vi "Graph vindu settinger.vi"(1 "Action(GET)":enum16{"GET", "SET"}(ring), 7 "Settigner fra MAin in":T1 {"Plot  L1"."Line Width" items=["0", "1", "2", "3", "4", "5"]; "Plot  L1"."Var Tag" items=["", "Wire Length", "Wire Tension", "Wire Speed", "Topside Voltage", "Tool Head Voltage", "Current", "Resistance"]; "Plot  L2"."Line Width" items=["0", "1", "2", "3", "4", "5"]; "Plot  L2"."Var Tag" items=["", "Wire Length", "Wire Tension", "Wire Speed", "Topside Voltage", "Tool Head Voltage", "Current", "Resistance"]; "Plot  R1"."Line Width" items=["0", "1", "2", "3", "4", "5"]; "Plot  R1"."Var Tag" items=["", "Wire Length", "Wire Tension", "Wire Speed", "Topside Voltage", "Tool Head Voltage", "Current", "Resistance"]; "Plot  R2"."Line Width" items=["0", "1", "2", "3", "4", "5"]; "Plot  R2"."Var Tag" items=["", "Wire Length", "Wire Tension", "Wire Speed", "Topside Voltage", "Tool Head Voltage", "Current", "Resistance"]}, 11 "error in (no error)":errorcluster) -> (8 "Settigner fra MAin out":T1 {"Plot  L1"."Line Width" items=["0", "1", "2", "3", "4", "5"]; "Plot  L1"."Var Tag" items=["", "Wire Length", "Wire Tension", "Wire Speed", "Topside Voltage", "Tool Head Voltage", "Current", "Resistance"]; "Plot  L2"."Line Width" items=["0", "1", "2", "3", "4", "5"]; "Plot  L2"."Var Tag" items=["", "Wire Length", "Wire Tension", "Wire Speed", "Topside Voltage", "Tool Head Voltage", "Current", "Resistance"]; "Plot  R1"."Line Width" items=["0", "1", "2", "3", "4", "5"]; "Plot  R1"."Var Tag" items=["", "Wire Length", "Wire Tension", "Wire Speed", "Topside Voltage", "Tool Head Voltage", "Current", "Resistance"]; "Plot  R2"."Line Width" items=["0", "1", "2", "3", "4", "5"]; "Plot  R2"."Var Tag" items=["", "Wire Length", "Wire Tension", "Wire Speed", "Topside Voltage", "Tool Head Voltage", "Current", "Resistance"]}, 15 "error out":errorcluster)   [LabVIEW 2011]
uses:
  Settigner fra Main.ctl
  Graph/Plot selector.ctl
  Graph/Y scale cluster.ctl
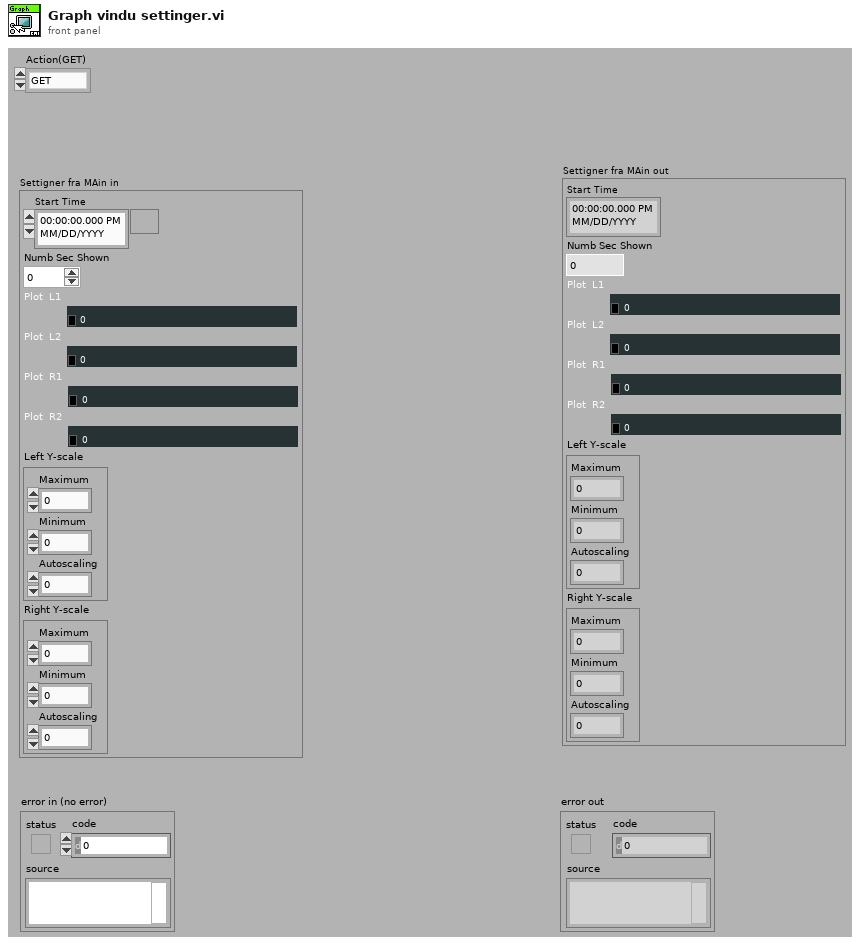
[diagram p1: front panel]
types:
  T1 = typedef "Settigner fra Main.ctl" = cluster{"Start Time":timestamp, "Numb Sec Shown":i32, "Plot  L1":T2, "Plot  L2":T2, "Plot  R1":T2, "Plot  R2":T2, "Left Y-scale":T3, "Right Y-scale":T3}
  T2 = typedef "Plot selector.ctl" = cluster{"Var Tag":u16, "Color":u32, "Line Width":u16}
  T3 = typedef "Y scale cluster.ctl" = cluster{"Maximum":dbl, "Minimum":dbl, "Autoscaling":i32}
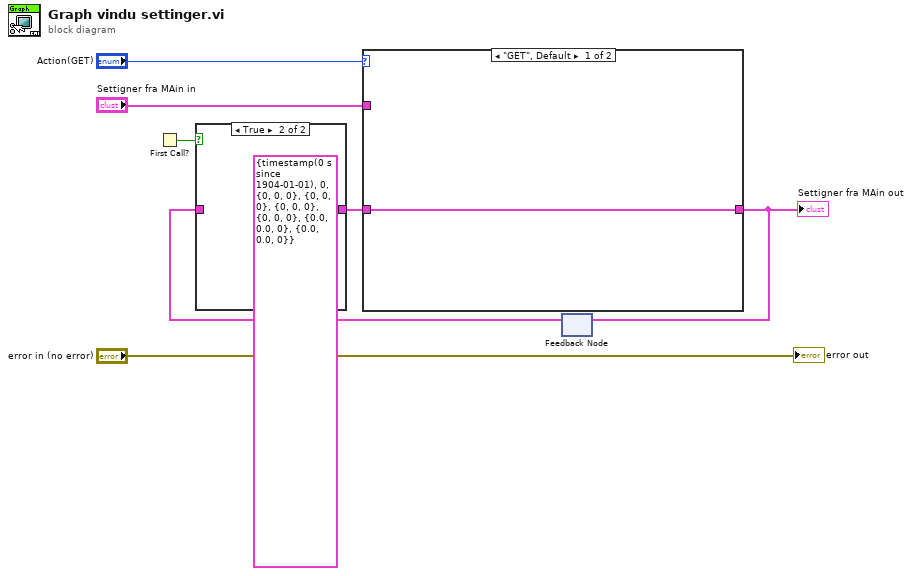
[diagram p0: block diagram]
diagram:
  n1 = First Call?() -> (First Call?: T/F=w4:bool)
  n2 = feedback #1() -> (w5:T1)  [unwired: 1 in]
  n3 = case shown="True" w4 {
    tunnel: w5 -> [w8 _]
    tunnel: [w8 T1 {"Start Time"=timestamp(0 s since 1904-01-01), "Numb Sec Shown"=0, "Plot  L1"={"Var Tag"=0, "Color"=0, "Line Width"=0}, "Plot  L2"={"Var Tag"=0, "Color"=0, "Line Width"=0}, "Plot  R1"={"Var Tag"=0, "Color"=0, "Line Width"=0}, "Plot  R2"={"Var Tag"=0, "Color"=0, "Line Width"=0}, "Left Y-scale"={"Maximum"=0.0, "Minimum"=0.0, "Autoscaling"=0}, "Right Y-scale"={"Maximum"=0.0, "Minimum"=0.0, "Autoscaling"=0}} ("Settigner fra MAin")] -> w2
    frame False {
    }
    frame True {
    }
  }
  n4 = case shown="\"GET\", Default" "Action(GET)" {
    tunnel: [w10 w11] -> w3
    tunnel: w2 -> [w10 _]
    tunnel: "Settigner fra MAin in" -> [_ w11]
    frame "GET", Default {
    }
    frame "SET" {
    }
  }
  "Settigner fra MAin out" <- w3
  n5 = feedback-in #1(w3) -> ()
  "error out" <- "error in (no error)"
